vi "模板匹配.vi"() -> ()   [LabVIEW 2018]
uses:
  <vilib>/vision/NI_Vision_Development_Module.lvlib
  <vilib>/vision/Pattern Matching.llb/IMAQ Pattern Match All Advanced Options.ctl
  <vilib>/vision/Pattern Matching.llb/IMAQ Match Range Setting.ctl
panel:
  out "Image":T1(plugin-control)
  in  "学习模板":bool
  in  "载入图片":bool
  in  "匹配":bool
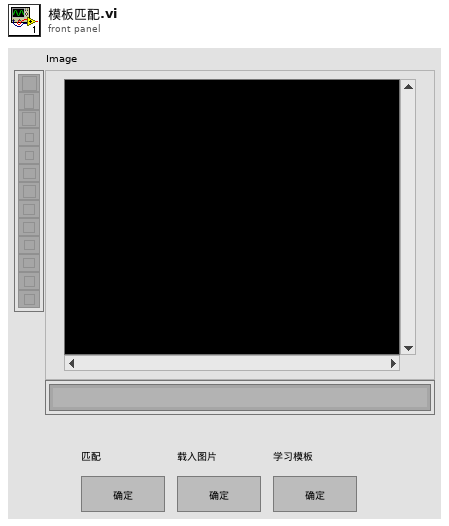
[diagram p1: front panel]
types:
  T1 = typedef "IMAQ Image.ctl" = refnum<image>
  T2 = typedef "IMAQ Match Range Setting.ctl" = cluster{"Match Constraints":u32, "Min":dbl, "Max":dbl}
  T3 = typedef "IMAQ Pattern Match All Advanced Options.ctl" = u16
  T4 = cluster{"Rotation":bool, "Scale":bool, "Occlusion":bool, "Reserved":bool, "Reserved":bool, "Reserved":bool}
  T5 = typedef "Image Type" = u32
  T6 = cluster{"Setup Data Item":u16, "Item Value":dbl}[]
  T7 = cluster{"Global Rectangle":i32[], "Contours":cluster{"Contour Type":u32, "ROI Type":u32, "Points":i32[]}[]}
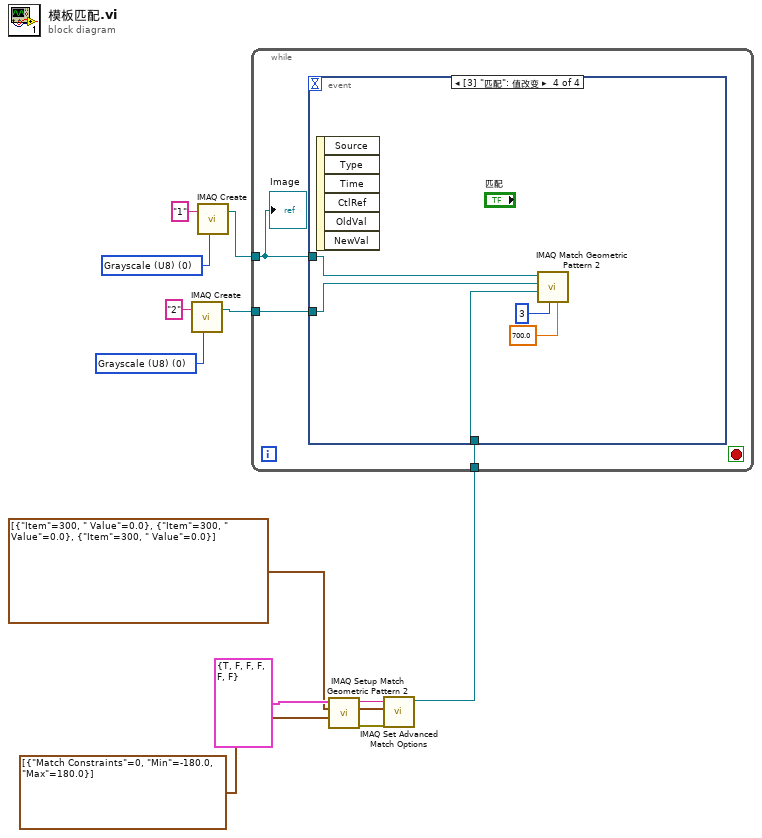
[diagram p0: block diagram]
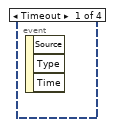
[diagram p2: hidden frame]
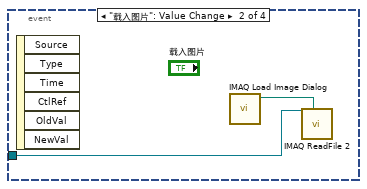
[diagram p3: hidden frame]
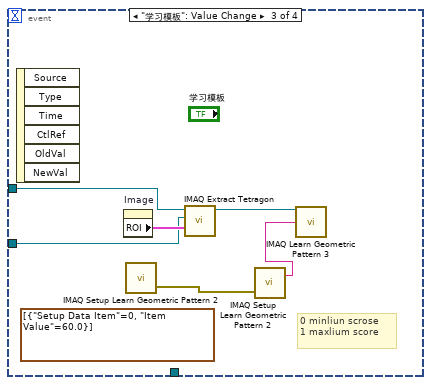
[diagram p4: hidden frame]
diagram:
  w8 = T5 0 items=["Grayscale (U8)", "Grayscale (I16)", "Grayscale (SGL)", "Complex (CSG)", "RGB (U32)", "HSL (U32)", "RGB (U64)", "Grayscale (U16)"] ("Image Type")
  w11 = T5 0 items=["Grayscale (U8)", "Grayscale (I16)", "Grayscale (SGL)", "Complex (CSG)", "RGB (U32)", "HSL (U32)", "RGB (U64)", "Grayscale (U16)"] ("Image Type")
  n1 = call "IMAQ Create"("Image Name"="2", "Image Type"=w8) -> ("New Image"=w7:T1)  [unwired: 3 in, 1 out]
  n2 = call "IMAQ Create"("Image Name"="1", "Image Type"=w11) -> ("New Image"=w10:T1)  [unwired: 3 in, 1 out]
  n3 = call "IMAQ Setup Match Geometric Pattern 2"("Range Settings"=T2[] [{"Match Constraints"=0, "Min"=-180.0, "Max"=180.0}], "Match Mode"=T4 {"Rotation"=TRUE, "Scale"=FALSE, "Occlusion"=FALSE, "Reserved"=FALSE, "Reserved"=FALSE, "Reserved"=FALSE}) -> ("error out"=w6:errorcluster, "Match Geometric Pattern 2 Setup Data"=w5:string)  [unwired: 8 in]
  n4 = call "IMAQ Set Advanced Match Options"("error in (no error)"=w6, "Advanced Match Options"=cluster{"Item":T3, " Value":dbl}[] [{"Item"=300, " Value"=0.0}, {"Item"=300, " Value"=0.0}, {"Item"=300, " Value"=0.0}], "Template In"=w5) -> ("Template Out"=w1:T1)  [unwired: 7 in, 1 out]
  n5 = while {
    tunnel: w10 -> [w15]
    tunnel: w7 -> [w14]
    tunnel: w1 -> [w13]
    stop <- _ stop-if-true
    n6 = event shown="[3] \"匹配\": 值改变" {
      selector: _ -> [_ _ _ _]
      dyn-events: _ -> [_ _ _ _]
      timeout: _ -> [_ _ _ _]
      tunnel: w15 -> [_ w16 w23 w28]
      tunnel: w14 -> [_ _ w22 w27]
      tunnel: w13 -> [_ _ _ w29]
      event Timeout {
        n7 = event-data() -> ()  [unwired: 1 in, 3 out]
      }
      event "载入图片": Value Change {
        n8 = event-data() -> ()  [unwired: 1 in, 6 out]
        n9 = call "IMAQ Load Image Dialog"() -> ("Path"=w17:path)  [unwired: 9 in, 2 out]
        n10 = call "IMAQ ReadFile 2"("File Path"=w17, "Image"=w16) -> ()  [unwired: 5 in, 5 out]
      }
      event "学习模板": Value Change {
        w18 = T6 [{"Setup Data Item"=0, "Item Value"=60.0}] ("Advanced Contour Match Options")
        # "0 minliun scrose\n1 maxlium score"
        n11 = event-data() -> ()  [unwired: 1 in, 6 out]
        n12 = property on="Image" class="ImageControl"() -> ("ROI"=w24:T7)  [unwired: 2 in, 2 out]
        n13 = call "IMAQ Setup Learn Geometric Pattern 2"() -> ("error out"=w20:errorcluster)  [unwired: 2 in, 1 out]
        n14 = call-poly "IMAQ Extract Tetragon"("ROI Descriptor"=w24, "Image Dst"=w22, "Image Src"=w23) -> ("Image Dst Out"=w21:T1)  [unwired: 7 in, 1 out]
        n15 = call "IMAQ Setup Learn Geometric Pattern 2"("error in (no error)"=w20) -> ("Learn Geometric Pattern 2 Setup Data"=w19:string)  [unwired: 1 in, 1 out]
        n16 = call "IMAQ Learn Geometric Pattern 3"("Template Image"=w21, "Learn Mask"=w19) -> ()  [unwired: 12 in, 2 out]
      }
      event "匹配": Value Change {
        n17 = event-data() -> ()  [unwired: 1 in, 6 out]
        n18 = call "IMAQ Match Geometric Pattern 2"("Minimum Match Score"=sgl 700.0, "Number of Matches Requested"=3, "Match Geometric Pattern 2 Setup Data"=w29, "Template Image"=w27, "Image"=w28) -> ()  [unwired: 3 in, 4 out]
      }
    }
    "Image" <- w15
  }
